vi "NoticeSmallStep.vi"(0 "array":dbl[](array[numeric]), 1 "previous index":i32, 2 "next index":i32, 3 "step size":i32, 4 "range size":i32) -> ()   [LabVIEW 2014]
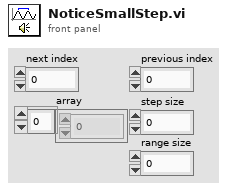
[diagram p1: front panel]
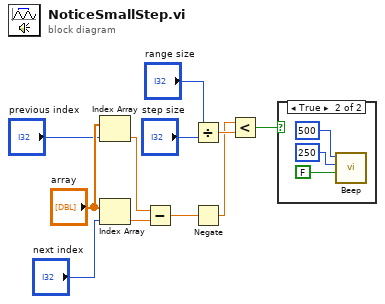
[diagram p0: block diagram]
diagram:
  n1 = Index Array(array="array", index="previous index") -> (element=w3:dbl)
  n2 = Index Array(array="array", index="next index") -> (element=w4:dbl)
  n3 = Subtract(x=w3, y=w4) -> (x-y=w9:dbl)
  n4 = Divide(x="range size", y="step size") -> (x/y=w11:dbl)
  n5 = Negate(x=w9) -> (-x=w8:dbl)
  n6 = Less?(x=w8, y=w11) -> (x < y?=w10:bool)
  n7 = case shown="True" w10 {
    frame False {
    }
    frame True {
      n8 = call <vilib>:"Beep.vi"("use system alert? (T)"=FALSE, "duration (msec)"=u32 250, "frequency (Hz)"=u32 500) -> ()  [unwired: 9 in]
    }
  }
